vi "PH_PPMA_PowerUnit.PC_StateTrigger.vi"(0 "i ref in":refnum<vi>, 2 "State Trigger":T1 caption="Enabling State" items=["no info", "off/false/out", "on/true/in", "Failure", "Alarm", "Status 1", "Status 2", "Status 3"], 3 "not linked?":bool, 5 "error in (no error)":errorcluster) -> (14 "i ref out":refnum<vi> caption="VI Refnum", 19 "error out":errorcluster)   [LabVIEW 2014, in "PH_PPMA_PowerUnit.lvlib"]
doc: "This VI writes the Trigger Tag Information to own attributes and sets the GUI object."
uses:
  PH_PPMA_PowerUnit.lvlib
  PH_Basics/PH_StatusHandler/PH_StatusHandler.Status.ctl
  PH_Basics/PH_Common/PH_Common.lvlib
  CS_Core/BaseSM/BaseSM.lvlib
  PH_Basics/PH_StatusHandler/PH_StatusHandler.lvlib
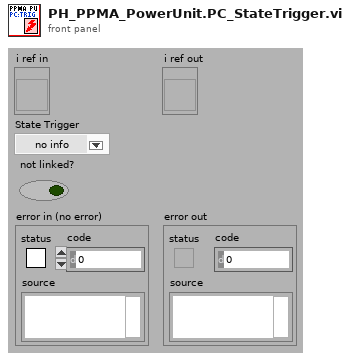
[diagram p1: front panel]
types:
  T1 = typedef "PH_StatusHandler.lvlib/PH_StatusHandler.Status.ctl" = i16
  T2 = typedef "PH_PPMA_PowerUnit.lvlib/PH_PPMA_PowerUnit.i attribute.ctl" = cluster{"GUI Refs":cluster{"Rods":refnum<vi>, "Ignitron":refnum<vi>, "Rossrelais":refnum<vi>, "Set Voltage":refnum<vi>, "PSU":refnum<vi>, "EOC":refnum<vi>, "Trigger":refnum<vi>}, "Rods":T3, "PSU":T4, "Ross Relais":T5, "Ignitron":T6, "Trigger":cluster{"State Device":T1, "linked?":bool}, "Timing Settings":cluster{"Prdc Fast?":bool, "Default Value Periodic Interval":i32, "Mercury on since":dbl, "Warm up Time Mercury [s]":dbl}, "Set Voltage [V]":dbl}
  T3 = typedef "PH_PPMA_PowerUnit.lvlib/PH_PPMA_PowerUnit.Rods Attributes.ctl" = cluster{"Instancename":string, "Device Status":T1, "linked?":bool}
  T4 = typedef "PH_PP_Common.lvlib/PH_PP_Common.PSU Attributes.ctl" = cluster{"lower limit [V]":dbl, "upper limit [V]":dbl, "Voltage set":bool, "State Device":T1, "linked?":bool}
  T5 = typedef "PH_PP_Common.lvlib/PH_PP_Common.Ross Relais Attributes.ctl" = cluster{"State Device":T1, "linked?":bool}
  T6 = typedef "PH_PP_Common.lvlib/PH_PP_Common.Ignitron Attributes.ctl" = cluster{"State Device":T1, "linked?":bool}
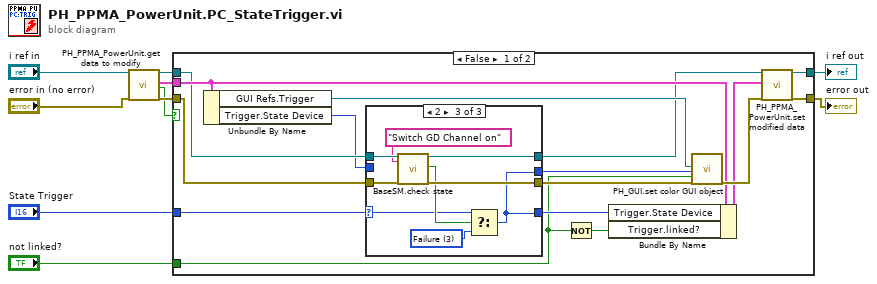
[diagram p0: block diagram]
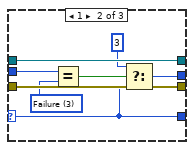
[diagram p3: hidden frame]
diagram:
  n1 = call "PH_PPMA_PowerUnit.get data to modify.vi"("i ref in"="i ref in", "error in (no error)"="error in (no error)") -> ("i ref out"=w6:refnum<vi>, "i attribute"=w4:T2, "timed out"=w3:bool, "error out"=w5:errorcluster)  [unwired: 14 in]
  n2 = case shown="False" w3 {
    tunnel: w6 -> [w22 w48]
    tunnel: [w12 w48] -> w9
    tunnel: w5 -> [w20 w47]
    tunnel: [w11 w47] -> w10
    tunnel: w4 -> [w23 _]
    tunnel: "State Trigger" -> [w15 _]
    tunnel: "not linked?" -> [w14 _]
    frame False {
      n3 = Unbundle By Name(w23) -> ("GUI Refs.Trigger"=w25:refnum<vi>, "Trigger.State Device"=w18:T1)
      n4 = case shown="2" w15 {
        selector: w15 -> [w29 w31 w39]
        tunnel: [w29 w31 w40] -> w17
        tunnel: [w29 w32 w40] -> w16
        tunnel: w20 -> [w27 w36 w44]
        tunnel: [w27 w36 w43] -> w19
        tunnel: w22 -> [w28 w37 w46]
        tunnel: [w28 w37 w45] -> w21
        tunnel: w18 -> [_ w35 _]
        frame 0, Default {
        }
        frame 1 {
          w30 = T1 3 items=["no info", "off/false/out", "on/true/in", "Failure", "Alarm", "Status 1", "Status 2", "Status 3"] ("Trigger.State Device")
          n5 = Equal?(x=w35, y=w30) -> (x = y?=w34:bool)
          n6 = Select(t=3, s=w34, f=w31) -> (s? t:f=w32:i32)
        }
        frame 2 {
          w38 = T1 3 items=["no info", "off/false/out", "on/true/in", "Failure", "Alarm", "Status 1", "Status 2", "Status 3"] ("Trigger.State Device")
          n7 = call "BaseSM.check state.vi"("i ref in"=w46, "requestedState"="Switch GD Channel on" ("requested state"), "error in (no error)"=w44) -> ("i ref out"=w45:refnum<vi>, "OK"=w41:bool, "error out"=w43:errorcluster)  [unwired: 11 in, 3 out]
          n8 = Select(t=w39, s=w41, f=w38) -> (s? t:f=w40:T1)
        }
      }
      n9 = Not(x=w14) -> (.not. x?=w13:bool)
      n10 = Bundle By Name(cluster=w23, "Trigger.State Device"=w17, "Trigger.linked?"=w13) -> (w24:T2)
      n11 = call "PH_GUI.set color GUI object.vi"("GUI object Ref"=w25, "State"=w16, "Blinking? (false)"=w14, "error in (no error)"=w19) -> ("error out"=w26:errorcluster)  [unwired: 15 in]
      n12 = call "PH_PPMA_PowerUnit.set modified data.vi"("i ref in"=w21, "i attribute"=w24, "error in (no error)"=w26) -> ("i ref out"=w12:refnum<vi>, "error out"=w11:errorcluster)  [unwired: 15 in]
    }
    frame True {
    }
  }
  "error out" <- w10
  "i ref out" <- w9
